vi "Demo_Andon get max ID with Breakdwn ID.vi"(7 "error in (no error)":errorcluster, 8 "Station No.":string, 9 "BREAKDOWN ID":i32, 10 "Refnum in":T1) -> (0 "error out":errorcluster, 1 "TABLE NAME":string, 2 "MAX BREAKDOWN ID":i32, 3 "Refnum out":T1, 4 "CONDITION string":string)   [LabVIEW 2017]
uses:
  <vilib>/addons/database/Connection.llb/Conn ObjectReference.ctl
  <vilib>/addons/database/Connection.llb/Conn Execute.vi
  <vilib>/addons/database/Recordset.llb/Rec Fetch Recordset Data (R).vi
  <vilib>/addons/database/Recordset.llb/Rec Destroy - Connection.vi
  <vilib>/addons/database/NI_Database_API.lvlib
panel:
  out "resulting string":string
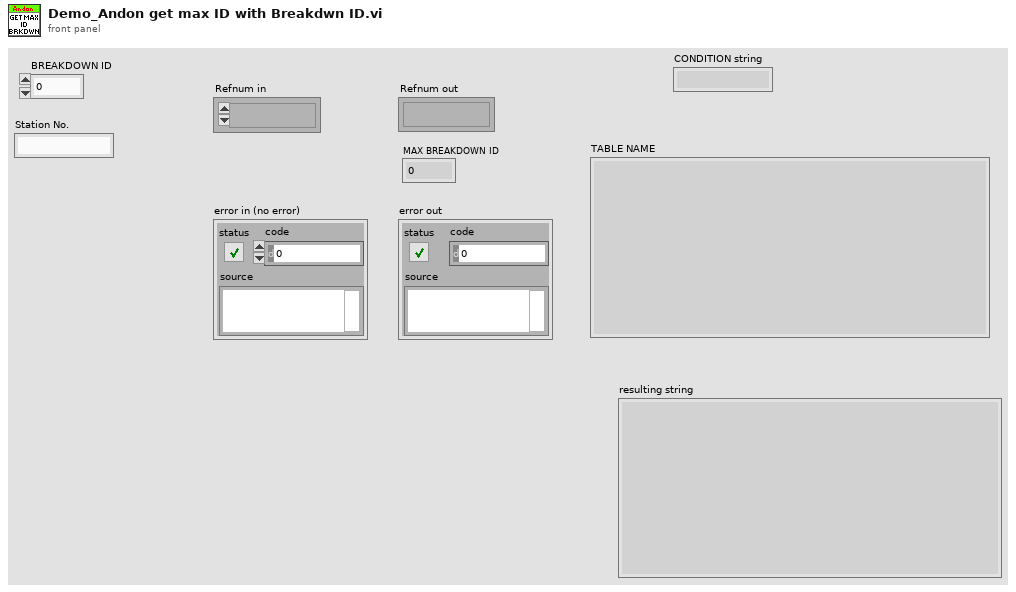
[diagram p1: front panel]
types:
  T1 = typedef "NI_Database_API.lvlib/Conn ObjectReference.ctl" = refnum<k1>
  T2 = typedef "NI_Database_API.lvlib/Rec ObjectReference.ctl" = refnum<k1>
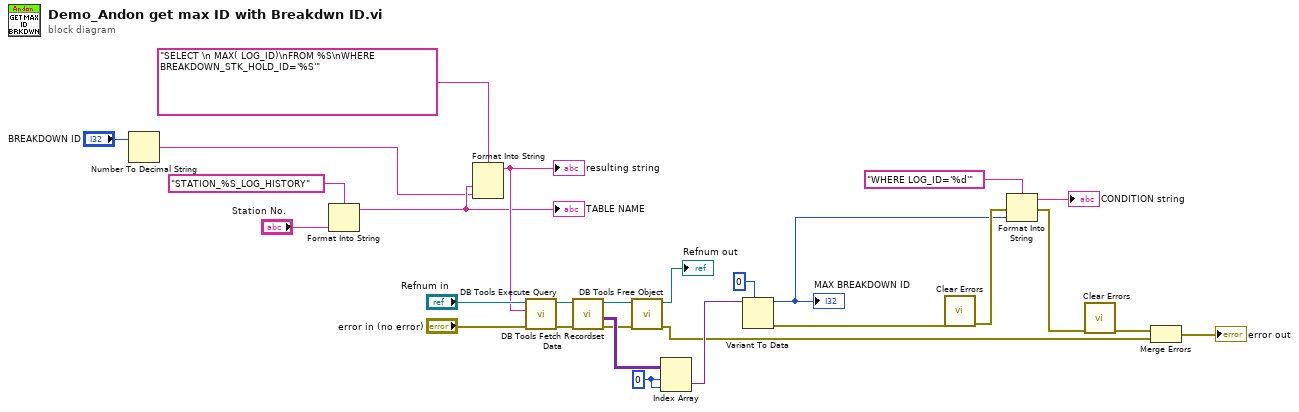
[diagram p0: block diagram]
diagram:
  w16 = 0 ("index (row)")
  n1 = Number To Decimal String(number="BREAKDOWN ID") -> (decimal integer string=w2:string)  [unwired: 1 in]
  n2 = Format Into String(format string="STATION_%S_LOG_HISTORY" ("SQL query"), "Station No.") -> (resulting string=w11:string)  [unwired: 2 in, 1 out]
  "TABLE NAME" <- w11
  n3 = Format Into String(format string="SELECT \n MAX( LOG_ID)\nFROM %S\nWHERE  BREAKDOWN_STK_HOLD_ID='%S'" ("SQL query"), w11, w2) -> (resulting string=w14:string)  [unwired: 2 in, 1 out]
  "resulting string" <- w14
  n4 = call-poly <vilib>:"DB Tools Execute Query.vi"("error in (no error)"="error in (no error)", "SQL query"=w14, "connection reference"="Refnum in") -> ("error out"=w20:errorcluster, "recordset reference"=w21:T2)  [unwired: 5 in]
  n5 = call-poly <vilib>:"DB Tools Fetch Recordset Data.vi"("error in (no error)"=w20, "recordset reference"=w21) -> ("error out"=w19:errorcluster, "recordset data"=w23:variant[][], "recordset reference out"=w22:T2)  [unwired: 3 in]
  n6 = call-poly <vilib>:"DB Tools Free Object.vi"("error in (no error)"=w19, "recordset reference"=w22) -> ("error out"=w5:errorcluster, "connection reference"=→"Refnum out":T1)  [unwired: 8 in]
  n7 = Index Array(array=w23, index (row)=w16, index (col)=w16) -> (element=w17:variant)
  n8 = Variant To Data(type=0, Variant=w17) -> (data=w7:i32, error out=w27:errorcluster)  [unwired: 1 in]
  "MAX BREAKDOWN ID" <- w7
  n9 = call <vilib>:"Clear Errors.vi"("error in (no error)"=w27) -> ("error out"=w9:errorcluster)  [unwired: 5 in, 1 out]
  n10 = Format Into String(format string="WHERE LOG_ID='%d'" ("String"), error in=w9, w7) -> (resulting string=→"CONDITION string":string, error out=w4:errorcluster)  [unwired: 1 in]
  n11 = call <vilib>:"Clear Errors.vi"("error in (no error)"=w4) -> ("error out"=w3:errorcluster)  [unwired: 5 in, 1 out]
  n12 = Merge Errors(w3, w5) -> (→"error out":errorcluster)
